vi "Initialize Waveform TDMS Log File.vi"(8 "error in (no error)":errorcluster, 9 "Operation":T1, 10 "File Path":path, 11 "Waveform TDMS Log File Specification in":refnum<class "Waveform TDMS Log File Specification.lvclass">) -> (0 "error out":errorcluster, 1 "Log File out":refnum<class "Log File.lvclass">, 3 "Waveform TDMS Log File Specification out":refnum<class "Waveform TDMS Log File Specification.lvclass">)   [LabVIEW 2015, in "Waveform Data Logger Shared.lvlib" / "Waveform TDMS Log File Specification.lvclass"]
uses:
  Waveform TDMS Log File Specification.lvclass
  Engine/Classes/Logs/Log Files/Log File/Operation.ctl
  Engine/Classes/Logs/Log Files/Log File/Log File.lvclass
  Engine/Classes/Logs/Log Files/TDMS Log File/TDMS Log File.lvclass
  Log File Specification/Log File Specification.lvclass/Log File Specification.ctl
  TDMS Log File Specification/TDMS Log File Specification.lvclass/TDMS Log File Specification.ctl
  Engine/Classes/Logs/Log Files/TDMS Log File/TDMS Log File.lvclass/TDMS Log File.ctl
  Waveform TDMS Log File Specification.lvclass/Waveform TDMS Log File Specification.ctl
  Log File Specification/Log File Specification.lvclass
  TDMS Log File Specification/TDMS Log File Specification.lvclass
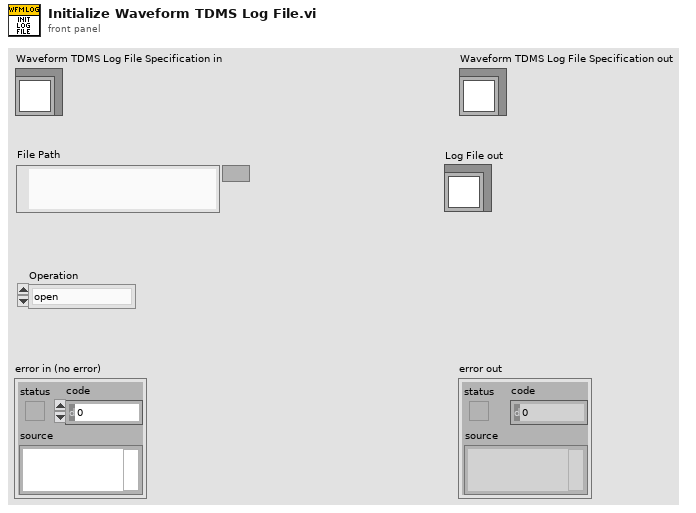
[diagram p1: front panel]
types:
  T1 = typedef "Waveform Data Logger Engine.lvlib/Log File.lvclass/Operation.ctl" = enum16{"open", "open or create", "create or replace", "create", "open (read-only)"}
  T2 = typedef "Waveform Data Logger Shared.lvlib/TDMS Log File Specification.lvclass/Property Specification.ctl" = cluster{"Name":string, "Value":variant}
  T3 = typedef "Waveform Data Logger Shared.lvlib/TDMS Log File Specification.lvclass/Channel Group Specification.ctl" = cluster{"Name":string, "Properties":T2[], "Channels":T4[]}
  T4 = typedef "Waveform Data Logger Shared.lvlib/TDMS Log File Specification.lvclass/Channel Specification.ctl" = cluster{"Name":string, "Properties":T2[]}
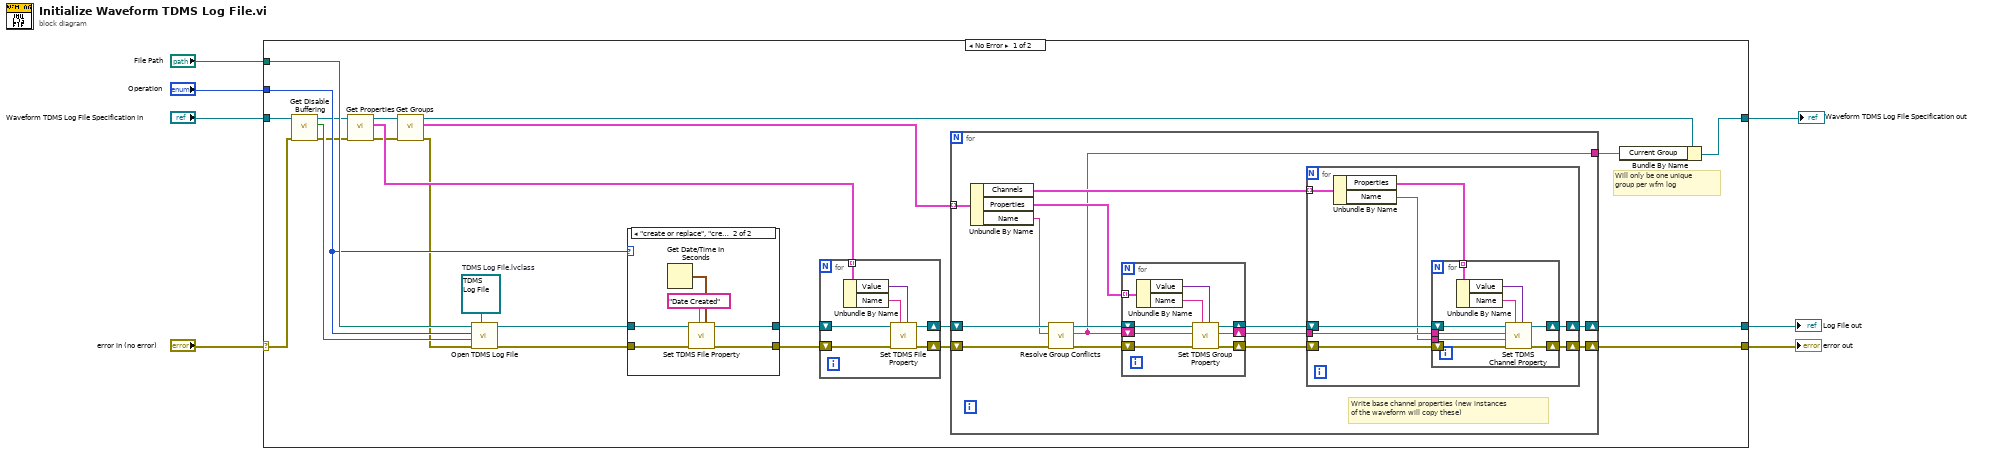
[diagram p0: block diagram]
diagram:
  n1 = case shown="No Error" "error in (no error)" {
    selector: "error in (no error)" -> [w31 w87]
    tunnel: [w9 w88] -> w3
    tunnel: "Waveform TDMS Log File Specification in" -> [w30 w88]
    tunnel: [w28 w87] -> w2
    tunnel: "File Path" -> [w26 _]
    tunnel: "Operation" -> [w18 _]
    tunnel: [w27 _] -> w1
    frame No Error {
      w25 = refnum<class "TDMS Log File.lvclass"> refnum  # TDMS Log File.lvclass
      # "Will only be one unique\ngroup per wfm log"
      n2 = call "Get Disable Buffering.vi"("error in (no error)"=w31, "Log File Specification in"=w30) -> ("error out"=w13:errorcluster, "Disable Buffering"=w29:bool, "Log File Specification out"=w17:refnum<class "Waveform TDMS Log File Specification.lvclass">)  [unwired: 7 in]
      n3 = call "Get Properties.vi"("error in (no error)"=w13, "TDMS Log File Specification in"=w17) -> ("error out"=w12:errorcluster, "Properties"=w16:T2[], "TDMS Log File Specification out"=w14:refnum<class "Waveform TDMS Log File Specification.lvclass">)  [unwired: 7 in]
      n4 = call "Get Groups.vi"("error in (no error)"=w12, "TDMS Log File Specification in"=w14) -> ("error out"=w11:errorcluster, "Groups"=w15:T3[], "TDMS Log File Specification out"=w10:refnum<class "Waveform TDMS Log File Specification.lvclass">)  [unwired: 7 in]
      n5 = call "Open TDMS Log File.vi"("TDMS Log File Type"=w25, "error in (no error)"=w11, "Disable Buffering (F)"=w29, "Operation"=w18, "File Path"=w26) -> ("error out"=w21:errorcluster, "TDMS Log File out"=w22:refnum<class "TDMS Log File.lvclass">)  [unwired: 5 in]
      n6 = case shown="\"create or replace\", \"create\"" w18 {
        tunnel: w22 -> [w33 w38]
        tunnel: w21 -> [w32 w37]
        tunnel: [w33 w36] -> w20
        tunnel: [w32 w35] -> w19
        frame Default {
        }
        frame "create or replace", "create" {
          n7 = Get Date/Time In Seconds() -> (seconds since 1Jan1904=w34:timestamp)
          n8 = call "Set TDMS File Property.vi"("Property Value"=w34, "Property Name"="Date Created" ("property names"), "error in (no error)"=w37, "TDMS Log File in"=w38) -> ("error out"=w35:errorcluster, "TDMS Log File out"=w36:refnum<class "TDMS Log File.lvclass">)  [unwired: 6 in]
        }
      }
      n9 = for {
        tunnel: w16 -> [w86] mode=indexing
        shift-right: [w85] -> w24
        shift-left: w20 -> [w84]
        shift-right: [w82] -> w23
        shift-left: w19 -> [w83]
        n10 = Unbundle By Name(w86) -> ("Value"=w80:variant, "Name"=w81:string)
        n11 = call "Set TDMS File Property.vi"("Property Value"=w80, "Property Name"=w81, "error in (no error)"=w83, "TDMS Log File in"=w84) -> ("error out"=w82:errorcluster, "TDMS Log File out"=w85:refnum<class "TDMS Log File.lvclass">)  [unwired: 6 in]
      }
      n12 = for {
        shift-right: [w49] -> w27
        shift-left: w24 -> [w46]
        shift-right: [w48] -> w28
        shift-left: w23 -> [w45]
        tunnel: w15 -> [w41] mode=indexing
        tunnel: [w40] -> w8
        # "Write base channel properties (new instances\nof the waveform will copy these)"
        n13 = Unbundle By Name(w41) -> ("Channels"=w52:T4[], "Properties"=w53:T2[], "Name"=w42:string)
        n14 = call "Resolve Group Conflicts.vi"("error in (no error)"=w45, "Group Name in"=w42, "TDMS Log File in"=w46) -> ("error out"=w44:errorcluster, "Group Name out"=w40:string, "TDMS Log File out"=w43:refnum<class "TDMS Log File.lvclass">)  [unwired: 5 in, 1 out]
        n15 = for {
          tunnel: w53 -> [w60] mode=indexing
          shift-right: [w59] -> w51
          shift-left: w43 -> [w62]
          shift-right: [w56] -> w47
          shift-left: w40 -> [w57]
          shift-right: [w58] -> w50
          shift-left: w44 -> [w61]
          n16 = Unbundle By Name(w60) -> ("Value"=w54:variant, "Name"=w55:string)
          n17 = call "Set TDMS Group Property.vi"("Property Value"=w54, "Property Name"=w55, "error in (no error)"=w61, "Group Name in"=w57, "TDMS Log File in"=w62) -> ("error out"=w58:errorcluster, "Group Name out"=w56:string, "TDMS Log File out"=w59:refnum<class "TDMS Log File.lvclass">)  [unwired: 4 in]
        }
        n18 = for {
          tunnel: w52 -> [w69] mode=indexing
          shift-right: [w64] -> w49
          shift-left: w51 -> [w68]
          shift-right: [w63] -> w48
          shift-left: w50 -> [w67]
          tunnel: w47 -> [w66]
          n19 = Unbundle By Name(w69) -> ("Properties"=w70:T2[], "Name"=w65:string)
          n20 = for {
            tunnel: w70 -> [w79] mode=indexing
            shift-right: [w74] -> w64
            shift-left: w68 -> [w78]
            shift-right: [w73] -> w63
            shift-left: w67 -> [w77]
            tunnel: w66 -> [w72]
            tunnel: w65 -> [w71]
            n21 = Unbundle By Name(w79) -> ("Value"=w76:variant, "Name"=w75:string)
            n22 = call "Set TDMS Channel Property.vi"("Property Value"=w76, "Property Name"=w75, "error in (no error)"=w77, "Channel Name in"=w71, "Group Name in"=w72, "TDMS Log File in"=w78) -> ("error out"=w73:errorcluster, "TDMS Log File out"=w74:refnum<class "TDMS Log File.lvclass">)  [unwired: 2 in, 2 out]
          }
        }
      }
      n23 = Bundle By Name(cluster=w10, "Current Group"=w8) -> (w9:refnum<class "Waveform TDMS Log File Specification.lvclass">)
    }
    frame Error {
    }
  }
  "error out" <- w2
  "Waveform TDMS Log File Specification out" <- w3
  "Log File out" <- w1
